vi "Validate Attributes JSON.vi"(6 "$Path":string="$.Attributes", 8 "error in":errorcluster, 10 "Cluster in":variant, 11 "<JSON>":string) -> (0 "error out":errorcluster, 2 "<JSON>":string)   [LabVIEW 2023]
uses:
  b690fbb4-b114-4137-a40c-faf688a51290.vi
  <vilib>/JDP Science/JSONtext/Next JSON Value.vi
  <vilib>/JDP Science/JSONtext/String Subset.vi
  <vilib>/JDP Science/JSONtext/Parsing/Advance past next JSON Value (inlined COPY).vi
  <vilib>/JDP Science/JSONtext/Parsing/Advance past whitespace.vi
  <vilib>/JDP Science/JSONtext/Parsing/Advance past String.vi
  <vilib>/JDP Science/JSONtext/Parsing/Advance past Number.vi
  <vilib>/JDP Science/JSONtext/Parsing/Advance past Line Ending.vi
  <vilib>/JDP Science/JSONtext/Variant to JSON Text.vi
  <vilib>/JDP Science/JSONtext/Parsing/Parse Full Path or Item Name.vi
  <vilib>/JDP Science/JSONtext/Parsing/Advance past Array.vi
  <vilib>/JDP Science/JSONtext/Parsing/Advance past Object.vi
  <vilib>/JDP Science/JSONtext/support/Error Cluster From Code.vi
  <vilib>/JDP Science/JSONtext/Offset/Find Item Locations by Path.vi
  <vilib>/JDP Science/JSONtext/LVClass Serializer/JSONtext LVClass Serializer.lvclass
  <vilib>/ErrorRing/Error Ring.xnode
  <vilib>/JDP Science/JSONtext/JSONtext.lvlib
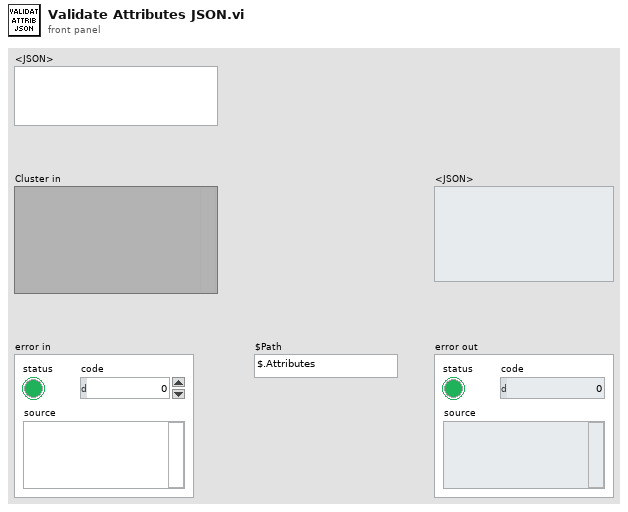
[diagram p1: front panel]
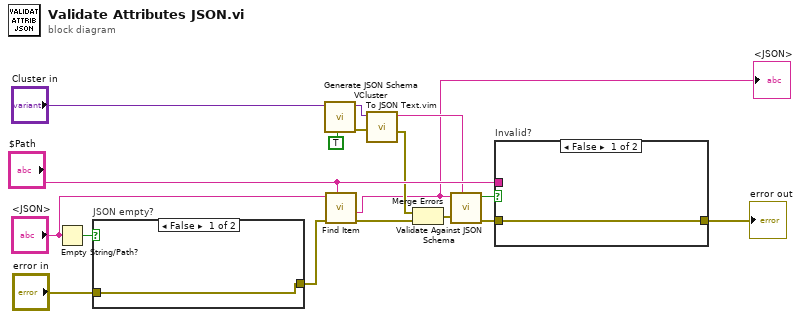
[diagram p0: block diagram]
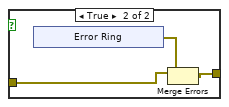
[diagram p2: hidden frame]
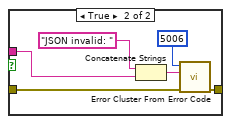
[diagram p3: hidden frame]
diagram:
  n1 = Empty String/Path?(string/path="<JSON>") -> (empty?=w4:bool)
  n2 = case "JSON empty?" shown="False" w4 {
    tunnel: "error in" -> [w18 w21]
    tunnel: [w18 w19] -> w2
    frame False {
    }
    frame True {
      n3 = xnode "Error Ring"() -> ("error out"=w20:errorcluster)
      n4 = Merge Errors(w21, w20) -> (w19:errorcluster)
    }
  }
  n5 = call "Generate JSON Schema VCluster.vi"("strict?"=TRUE, "type"="Cluster in") -> ("error out"=w8:errorcluster, "json schema cluster"=w7:variant)  [unwired: 8 in]
  n6 = call <vilib>:"Find Item.vi"("$Path or Item Name"="$Path", "error in (no error)"=w2, "JSON"="<JSON>") -> ("error out"=w13:errorcluster, "<JSON>"=w5:string)  [unwired: 5 in, 2 out]
  "<JSON>" <- w5
  n7 = call "To JSON Text.vim"("error in (no error)"=w8, "Anything"=w7) -> ("error out"=w10:errorcluster, "<JSON>"=w11:string)  [unwired: 8 in]
  n8 = Merge Errors(w10, w13) -> (w9:errorcluster)
  n9 = call <vilib>:"Validate Against JSON Schema.vi"("JSON Schema"=w11, "error in (no error)"=w9, "JSON"=w5) -> ("error out"=w14:errorcluster, "Invalid"=w16:bool)  [unwired: 4 in, 3 out]
  n10 = case "Invalid?" shown="False" w16 {
    tunnel: w14 -> [w27 w33]
    tunnel: [w27 w32] -> w15
    tunnel: "$Path" -> [_ w28]
    frame False {
    }
    frame True {
      n11 = Concatenate Strings("JSON invalid: " ("string"), w28) -> (w30:string)
      n12 = call <vilib>:"Error Cluster From Error Code.vi"("error in (no error)"=w33, "error message (\"\")"=w30, "error code (0)"=5006) -> ("error out"=w32:errorcluster)  [unwired: 6 in]
    }
  }
  "error out" <- w15
